vi "Trace Variable 1 hour Popup.vi"(11 "Tag":string="TNK1_Temperature") -> ()   [LabVIEW 2019]
uses:
  <vilib>/NI/AMC/Create Single Message.vi
  <vilib>/NI/AMC/Update Message Routing Info.vi
  <vilib>/NI/AMC/Read Termination Message.vi
  <vilib>/NI/AMC/Globals.vi
  <vilib>/NI/AMC/Send Message.vi
  <vilib>/NI/AMC/AMC.lvlib
panel:
  out "status":string
  in  "exit":bool
  out "TagName":string
  in  "Refresh Button":bool
  out "XY Graph":cluster{timestamp[], dbl[]}(graph)
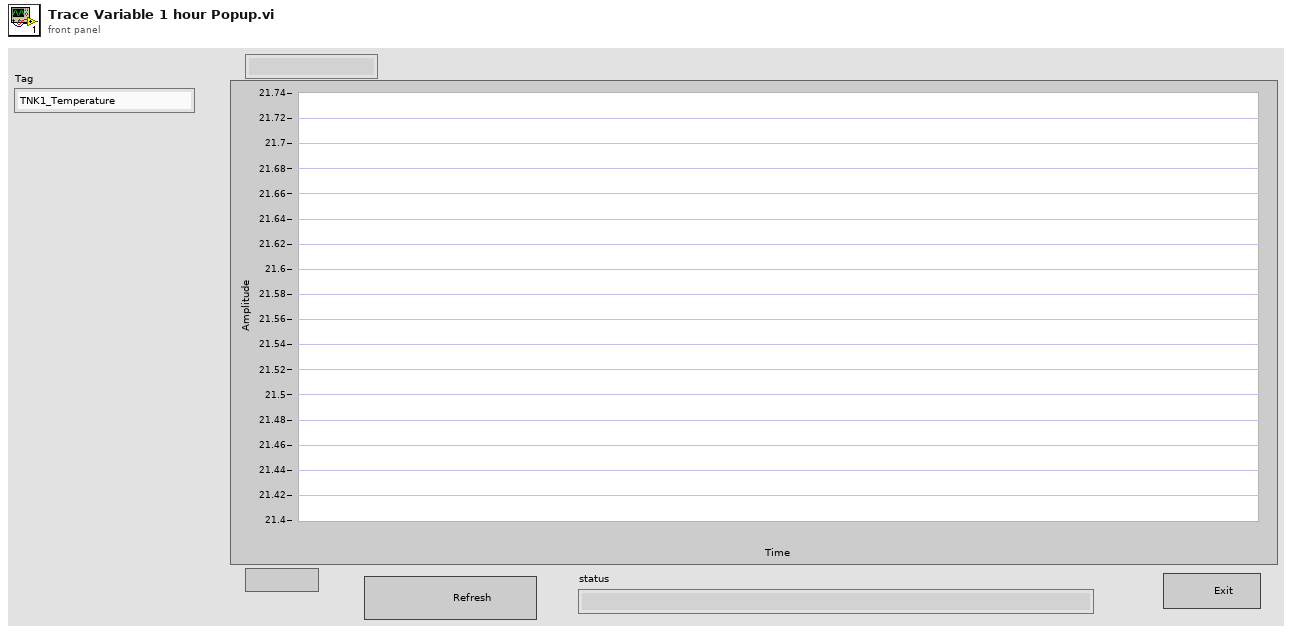
[diagram p1: front panel]
types:
  T1 = typedef "AMC.lvlib/Message Queue.ctl" = refnum<queue>
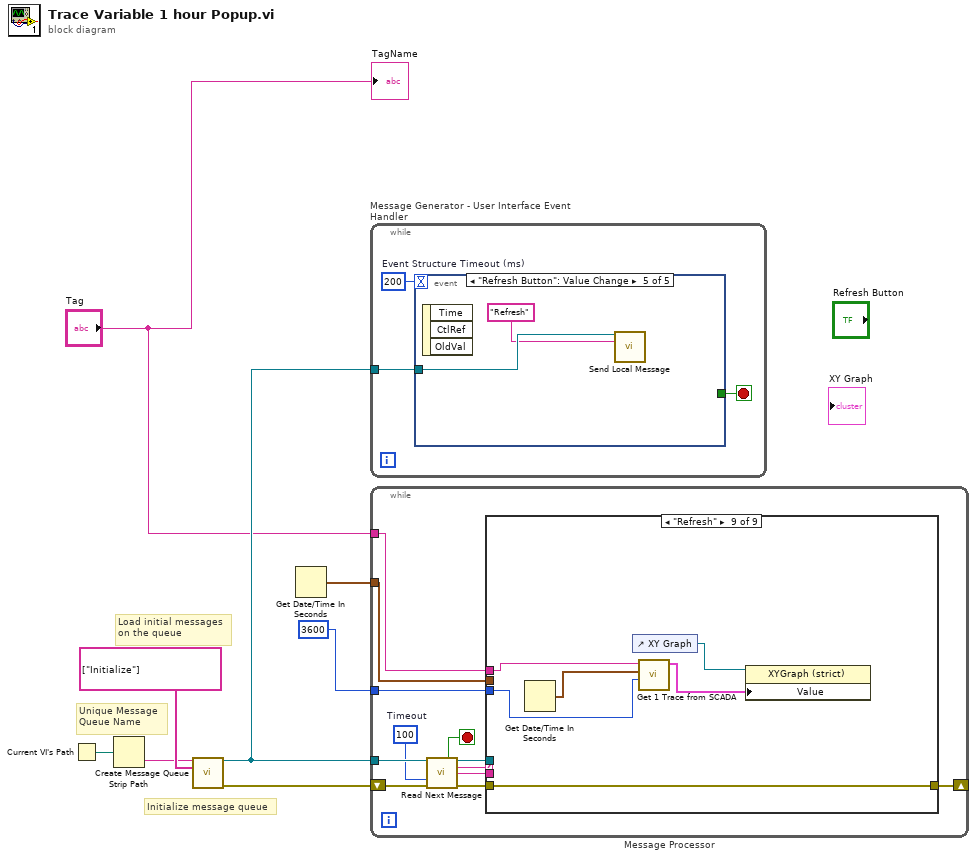
[diagram p0: block diagram]
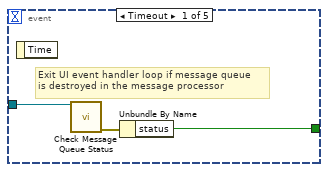
[diagram p2: hidden frame]
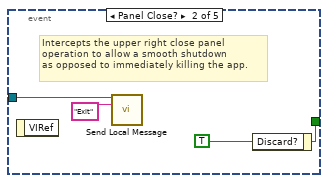
[diagram p3: hidden frame]
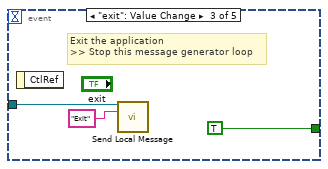
[diagram p4: hidden frame]
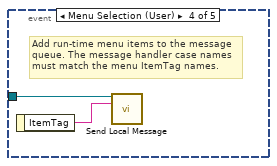
[diagram p5: hidden frame]
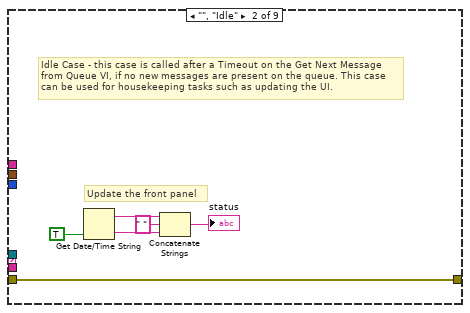
[diagram p7: hidden frame]
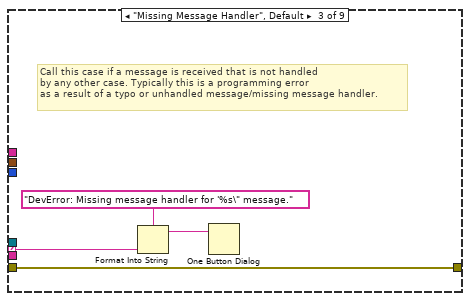
[diagram p8: hidden frame]
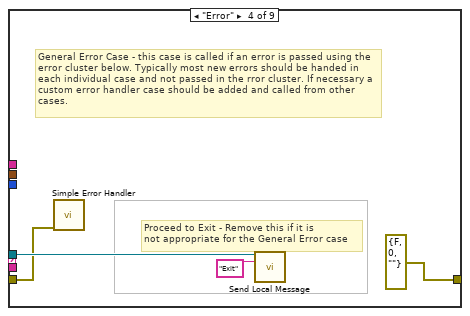
[diagram p9: hidden frame]
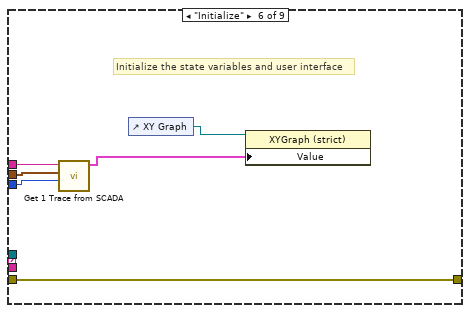
[diagram p11: hidden frame]
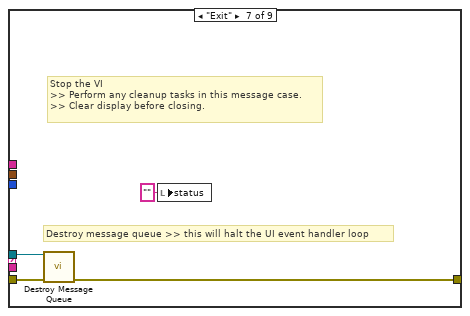
[diagram p12: hidden frame]
diagram:
  # "Initialize message queue"
  # "Unique Message\nQueue Name"
  # "Load initial messages\non the queue"
  n1 = Current VI's Path() -> (path=w4:path)
  n2 = Strip Path(path=w4) -> (name=w7:string)  [unwired: 1 out]
  n3 = call <vilib>:"Create Message Queue.vi"("message queue name"=w7, "initial message names"=string[] ["Initialize"]) -> ("message queue out"=w6:T1, "error out"=w5:errorcluster)  [unwired: 12 in]
  n4 = Get Date/Time In Seconds() -> (seconds since 1Jan1904=w2:timestamp)
  n5 = while "Message Generator - User Interface Event Handler" {
    tunnel: w6 -> [w9]
    stop <- w10 stop-if-true
    w11 = 200  # Event Structure Timeout (ms)
    n6 = event shown="[4] \"Refresh Button\": Value Change" {
      selector: _ -> [_ _ _ _ _]
      dyn-events: _ -> [_ _ _ _ _]
      timeout: w11 -> [_ _ _ _ _]
      tunnel: [w12 w17 TRUE ("Discard?") _ _] -> w10
      tunnel: w9 -> [w13 w15 w18 w21 w24]
      event Timeout {
        # "Exit UI event handler loop if message queue\nis destroyed in the message processor"
        n7 = event-data() -> ()  [unwired: 2 out]
        n8 = call <vilib>:"Check Message Queue Status.vi"("message queue in"=w13) -> ("error out"=w14:errorcluster)  [unwired: 10 in, 4 out]
        n9 = Unbundle By Name(w14) -> ("status"=w12:bool)
      }
      event Panel Close? {
        w17 = TRUE ("Discard?")
        # "Intercepts the upper right close panel\noperation to allow a smooth shutdown\nas opposed to immediately killing the app."
        n10 = event-data() -> ()  [unwired: 2 out]
        n11 = call <vilib>:"Send Local Message.vi"("message queue in"=w15, "message name"="Exit") -> ()  [unwired: 11 in, 3 out]
        n12 = event-data("Discard?"=w17) -> ()  [unwired: 1 in, 1 out]
      }
      event "exit": Value Change {
        # "Exit the application\n>> Stop this message generator loop"
        n13 = event-data() -> ()  [unwired: 2 out]
        n14 = call <vilib>:"Send Local Message.vi"("message queue in"=w18, "message name"="Exit") -> ()  [unwired: 11 in, 3 out]
      }
      event Menu Selection (User) {
        # "Add run-time menu items to the message\nqueue. The message handler case names must match the menu ItemTag names."
        n15 = event-data() -> ("ItemTag"=w22:string)  [unwired: 1 out]
        n16 = call <vilib>:"Send Local Message.vi"("message queue in"=w21, "message name"=w22) -> ()  [unwired: 11 in, 3 out]
      }
      event "Refresh Button": Value Change {
        n17 = event-data() -> ()  [unwired: 4 out]
        n18 = call <vilib>:"Send Local Message.vi"("message queue in"=w24, "message name"="Refresh") -> ()  [unwired: 11 in, 3 out]
      }
    }
  }
  n19 = while "Message Processor" {
    shift-left: w5 -> [w32]
    shift-right: [w36] -> _
    tunnel: w6 -> [w33]
    tunnel: "Tag" -> [w27]
    tunnel: w2 -> [w26]
    tunnel: 3600 -> [w25]
    stop <- w35 stop-if-true
    w28 = 100  # Timeout
    n20 = call <vilib>:"Read Next Message.vi"("message queue in"=w33, "timeout (1 ms)"=w28, "error in"=w32) -> ("exit process?"=w35:bool, "message queue out"=w34:T1, "message name"=w30:string, "message value"=w29:string, "error out"=w31:errorcluster)  [unwired: 5 in, 3 out]
    n21 = case shown="\"Refresh\"" w30 {
      selector: w30 -> [_ _ w46 _ _ _ _ _ _]
      tunnel: w34 -> [_ _ _ w50 _ _ w60 _ _]
      tunnel: w31 -> [w37 w43 w47 w48 w52 w58 w61 w63 w69]
      tunnel: [w37 w43 w47 errorcluster {"status"=FALSE, "code"=0, "source"=""} ("error out") w52 w58 w59 w63 w69] -> w36
      tunnel: w29 -> [_ _ _ _ _ _ _ _ _]
      tunnel: w27 -> [_ _ _ _ _ w55 _ _ w68]
      tunnel: w26 -> [_ _ _ _ _ w54 _ _ _]
      tunnel: w25 -> [_ _ _ _ _ w53 _ _ w66]
      frame "---------- Framework Operations ----------" {
        # "Dummy case to add a seperator in the Case Structure menu"
      }
      frame "", "Idle" {
        # "Update the front panel"
        # "Idle Case - this case is called after a Timeout on the Get Next Message from Queue VI, if no new messages are present on the queue. This case can be used for housekeeping tasks such as updating the UI."
        n22 = Get Date/Time String(want seconds? (F)=TRUE) -> (date string=w42:string, time string=w41:string)  [unwired: 2 out]
        n23 = Concatenate Strings(w42, " " ("string"), w41) -> (→"status":string)
      }
      frame "Missing Message Handler", Default {
        # "Call this case if a message is received that is not handled \nby any other case. Typically this is a programming error\nas a result of a typo or unhandled message/missing message handler."
        n24 = Format Into String(format string="DevError: Missing message handler for '%s\" message." ("message"), w46) -> (resulting string=w44:string)  [unwired: 2 in, 1 out]
        n25 = One Button Dialog(message=w44) -> ()  [unwired: 2 out]
      }
      frame "Error" {
        # "Proceed to Exit - Remove this if it is\nnot appropriate for the General Error case"
        # "General Error Case - this case is called if an error is passed using the error cluster below. Typically most new errors should be handed in each individual case and not passed in the rror cluster. If necessary a custom error handler case should be added and called from other cases."
        n26 = call <vilib>:"Simple Error Handler.vi"("error in (no error)"=w48) -> ()  [unwired: 1 in, 8 out]
        n27 = call <vilib>:"Send Local Message.vi"("message queue in"=w50, "message name"="Exit") -> ()  [unwired: 11 in, 3 out]
      }
      frame "---------- Generic Operations ----------" {
        # "Dummy case to add a seperator in the Case Structure menu"
      }
      frame "Initialize" {
        # "Initialize the state variables and user interface"
        n28 = call "Get 1 Trace from SCADA.vi"("Numeric"=w53, "seconds since 1Jan1904"=w54, "Tag"=w55) -> ("Cluster"=w56:cluster{timestamp[], dbl[]})  [unwired: 8 in]
        n29 = control-ref of="XY Graph"() -> (w57:refnum<vi>)
        n30 = property class="XYGraph (strict)"(reference=w57, "Value"=w56) -> ()  [unwired: 1 in, 2 out]
      }
      frame "Exit" {
        # "Destroy message queue >> this will halt the UI event handler loop"
        # "Stop the VI\n>> Perform any cleanup tasks in this message case.\n>> Clear display before closing."
        n31 = call <vilib>:"Destroy Message Queue.vi"("message queue in"=w60, "error in"=w61) -> ("error out"=w59:errorcluster)  [unwired: 11 in, 2 out]
        n32 = local write "status"("" ("Status")) -> ()
      }
      frame "---------- Application Operations ----------" {
      }
      frame "Refresh" {
        n33 = Get Date/Time In Seconds() -> (seconds since 1Jan1904=w67:timestamp)
        n34 = control-ref of="XY Graph"() -> (w65:refnum<vi>)
        n35 = call "Get 1 Trace from SCADA.vi"("Numeric"=w66, "seconds since 1Jan1904"=w67, "Tag"=w68) -> ("Cluster"=w64:cluster{timestamp[], dbl[]})  [unwired: 8 in]
        n36 = property class="XYGraph (strict)"(reference=w65, "Value"=w64) -> ()  [unwired: 1 in, 2 out]
      }
    }
  }
  "TagName" <- "Tag"
